vi "Call Helper to Run.vi"(11 "vi path":path) -> ()   [LabVIEW 2020, in "NI_TargetHelper.lvlib"]
uses:
  <vilib>/TargetSupport/NI_TargetHelper/NI_TargetHelper.lvlib
  <vilib>/TargetSupport/NI_TargetHelper/Instance VIref.ctl
  <vilib>/TargetSupport/NI_TargetHelper/Helper.vi
panel:
  out "error out":errorcluster
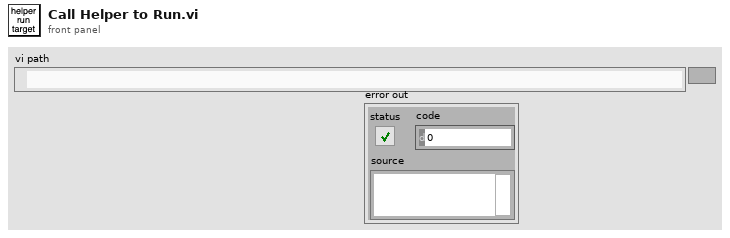
[diagram p1: front panel]
types:
  T1 = typedef "NI_TargetHelper.lvlib/Instance VIref.ctl" = refnum<vi>
  T2 = enum16{"status", "update", "compile", "deploy", "run", "stop"}
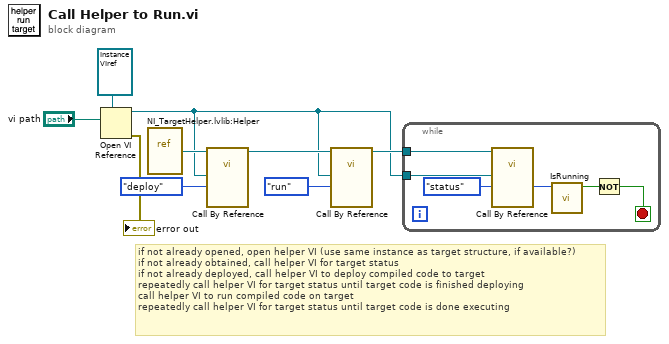
[diagram p0: block diagram]
diagram:
  # "if not already opened, open helper VI (use same instance as target structure, if available?)\nif not already obtained, call helper VI for target status\nif not already deployed, call helper VI to deploy compiled code to target\nrepeatedly call helper VI for target status until target code is finished deploying\ncall helper VI to run compiled code on target\nrepeatedly call helper VI for target status until target code is done executing"
  n1 = Open VI Reference(type specifier VI Refnum (for type only)=T1 refnum ("instVIref"), vi path="vi path") -> (vi reference=w4:T1, error out=→"error out":errorcluster)  [unwired: 4 in]
  n2 = vi-ref "NI_TargetHelper.lvlib:Helper.vi"() -> (w9:refnum<vi>)
  n3 = call-by-ref "?"(reference=w9, "op"=T2."deploy", "instVIref"=w4) -> (reference out=w7:refnum<vi>)  [unwired: 2 in, 2 out]
  n4 = call-by-ref "?"(reference=w7, "op"=T2."run", "instVIref"=w4) -> (reference out=w5:refnum<vi>)  [unwired: 2 in, 2 out]
  n5 = while {
    tunnel: w4 -> [w14]
    tunnel: w5 -> [w13]
    stop <- w10 stop-if-true
    n6 = call-by-ref "?"(reference=w13, "op"=T2."status", "instVIref"=w14) -> ("status"=w12:u64)  [unwired: 2 in, 2 out]
    n7 = call <vilib>:"IsRunning.vi"("status"=w12) -> ("running?"=w11:bool)  [unwired: 10 in]
    n8 = Not(x=w11) -> (.not. x?=w10:bool)
  }
